vi "tacking_math.vi"() -> (3 "Sailling Pts":cluster{"X":dbl, "Y":dbl}[](array[cluster]))   [LabVIEW 2013]
doc: "Calculates the nextoptimal tacking location, given:\n the waypoint and wind in the boat's frame of reference\n the maximum distance to travel before tacking\n the current estimated number of tacks needed to reach the waypoint\n and irons range\n\n(11/5/2014) Kaitlin Gallagher and Rocco Diverdi"
uses:
  <vilib>/Analysis/baseanly.llb/Real A x B.vi
  <vilib>/Analysis/NI_AALBase.lvlib
panel:
  in  "number of tacks":dbl
  out "Y":dbl
  out "X":dbl
  in  "Max Tack Length":dbl
  in  "Irons Range":dbl
  in  "Wind":dbl
  in  "Waypoint":cluster{"X":dbl, "Y":dbl}
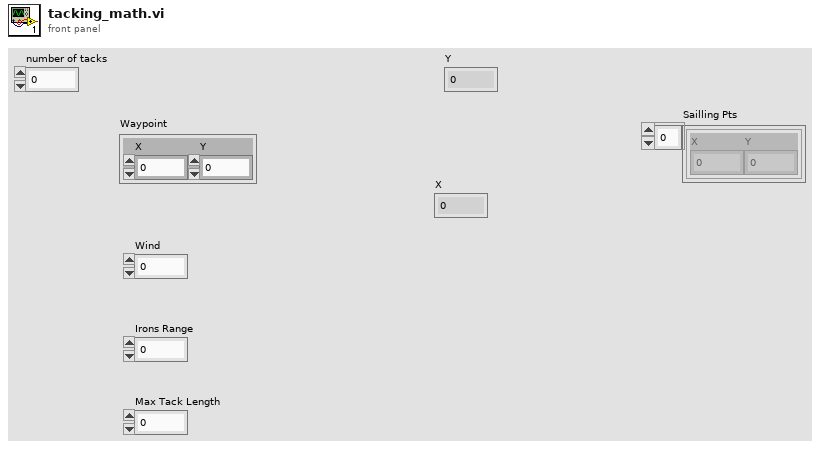
[diagram p1: front panel]
types:
  T1 = typedef "NI_Matrix.lvlib/RealMatrix.ctl" = dbl[][]
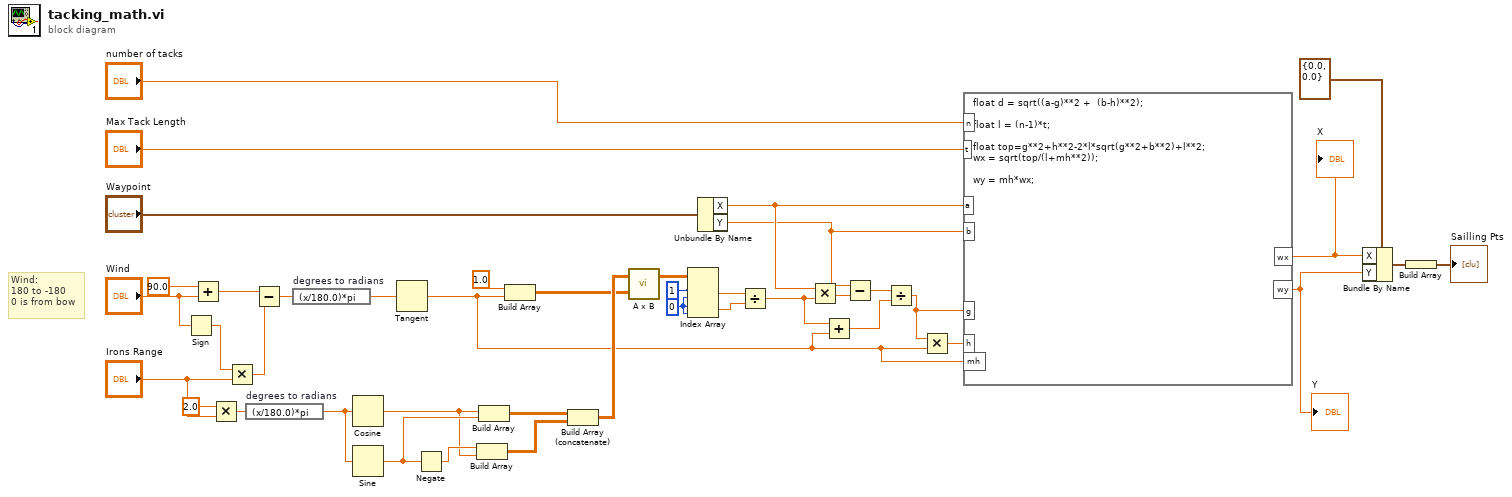
[diagram p0: block diagram]
diagram:
  w16 = 0 ("index (row)")
  # "Wind:\n180 to -180\n0 is from bow"
  n1 = Sign(1:"Wind") -> (0:w37:dbl)
  n2 = Add(x=90.0, y="Wind") -> (x+y=w39:dbl)
  n3 = Multiply(x=2.0, y="Irons Range") -> (x*y=w23:dbl)
  n4 = Multiply(x=w37, y="Irons Range") -> (x*y=w38:dbl)
  n5 = expression code="(x/180.0)*pi" "degrees to radians"(w23) -> (w22:dbl)
  n6 = Subtract(x=w39, y=w38) -> (x-y=w35:dbl)
  n7 = expression code="(x/180.0)*pi" "degrees to radians"(w35) -> (w34:dbl)
  n8 = Cosine(x=w22) -> (cos(x)=w28:dbl)
  n9 = Sine(x=w22) -> (sin(x)=w30:dbl)
  n10 = Tangent(1:w34) -> (0:w7:dbl)
  n11 = Negate(x=w30) -> (-x=w29:dbl)
  n12 = Build Array(w29, w28) -> (w26:T1)
  n13 = Build Array(w28, w30) -> (w27:T1)
  n14 = Build Array(1.0, w7) -> (w24:T1)
  n15 = Build Array (concatenate)(w27, w26) -> (w25:T1)
  n16 = call-poly <vilib>:"A x B.vi"("B"=w24, "A"=w25) -> ("A x B"=w21:T1)  [unwired: 1 out]
  n17 = Index Array(array=w21, index (row) #1=1 ("index (row)"), index (col) #1=w16, index (row) #2=w16, index (col) #2=w16) -> (element #1=w19:dbl, element #2=w18:dbl)
  n18 = Unbundle By Name("Waypoint") -> ("X"=w10:dbl, "Y"=w9:dbl)
  n19 = Divide(x=w19, y=w18) -> (x/y=w15:dbl)
  n20 = Multiply(x=w10, y=w15) -> (x*y=w17:dbl)
  n21 = Add(x=w15, y=w7) -> (x+y=w13:dbl)
  n22 = Subtract(x=w9, y=w17) -> (x-y=w14:dbl)
  n23 = Divide(x=w14, y=w13) -> (x/y=w11:dbl)
  n24 = Multiply(x=w11, y=w7) -> (x*y=w12:dbl)
  n25 = formula code="float d = sqrt((a-g)**2 +  (b-h)**2);\n\nfloat l = (n-1)*t;\n\nfloat top=g**2+h**2-2*l*sqrt(g**2+b**2)+l**2;\nwx = sqrt(top/(l+mh**2));\n\nwy = mh*wx;"("a"=w10, "b"=w9, "g"=w11, "h"=w12, "t"="Max Tack Length", "mh"=w7, "n"="number of tacks") -> ("wx"=w5:dbl, "wy"=w3:dbl)
  "X" <- w5
  "Y" <- w3
  n26 = Bundle By Name(cluster=cluster{"Y":dbl, "X":dbl} {"Y"=0.0, "X"=0.0} ("Waypoint"), "X"=w5, "Y"=w3) -> (w2:cluster{"Y":dbl, "X":dbl})
  n27 = Build Array(w2) -> (→"Sailling Pts":cluster{"Y":dbl, "X":dbl}[])
